vi "Save VIs in a Folder.vi"(8 "error in (no error)":errorcluster, 11 "VI Folder":path) -> (0 "error out":errorcluster, 3 "VI List":path[](array[path]))   [LabVIEW 2016, in "SLL Scripting.lvlib"]
doc: "This VI can be used to save the list of all VIs in a folder."
uses:
  SLL Scripting.lvlib
panel:
  out "Progress":i32
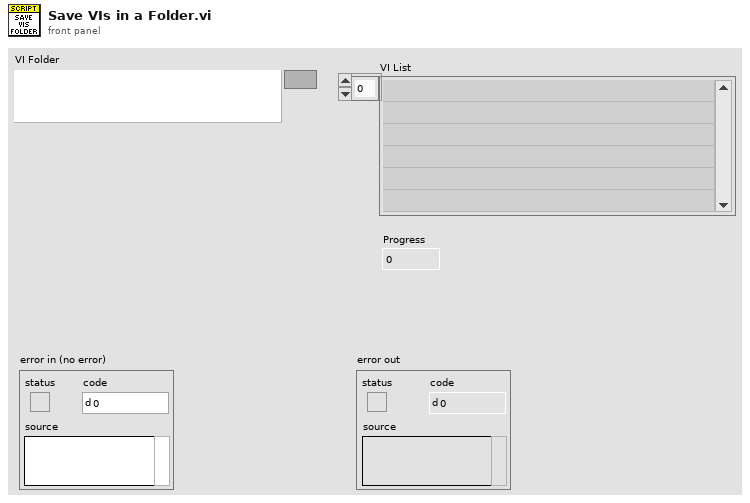
[diagram p1: front panel]
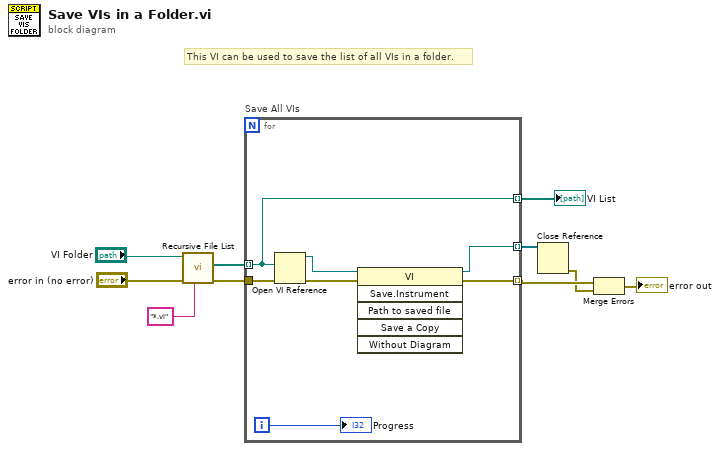
[diagram p0: block diagram]
diagram:
  # "This VI can be used to save the list of all VIs in a folder."
  n1 = call <vilib>:"Recursive File List.vi"("pattern"="*.vi", "error in (no error)"="error in (no error)", "Folder Path"="VI Folder") -> ("error out"=w4:errorcluster, "All Files in Dir"=w7:path[])  [unwired: 4 in, 3 out]
  n2 = for "Save All VIs" {
    tunnel: [w11] -> w10 mode=indexing
    tunnel: w7 -> [w17] mode=indexing
    tunnel: [w17] -> w6 mode=indexing
    tunnel: w4 -> [w16]
    tunnel: [w13] -> w3 mode=indexing
    i -> [w14]
    n3 = Open VI Reference(vi path=w17, error in (no error)=w16) -> (vi reference=w12:refnum<vi>, error out=w15:errorcluster)  [unwired: 4 in]
    n4 = invoke class="VI" method="Save.Instrument"(reference=w12, error in=w15) -> (reference out=w11:refnum<vi>, error out=w13:errorcluster)  [unwired: 4 in, 4 out]
    "Progress" <- w14
  }
  "VI List" <- w6
  n5 = Close Reference(reference=w10) -> (error out=w2:errorcluster)  [unwired: 1 in]
  n6 = Merge Errors(w3, w2) -> (→"error out":errorcluster)
